vi "Measure_Voltage.vi"(6 "Resolution in Digits":T1(ring), 8 "error in (no error)":errorcluster, 9 "Range":dbl=1.2, 10 "Level":dbl=1.2, 11 "NI-DCPower in":refnum<class "niDCPower.lvclass">) -> (0 "error out":errorcluster, 1 "Out of Range":bool, 2 "DC_Voltage":dbl, 3 "NI-DCPower out":refnum<class "niDCPower.lvclass">)   [LabVIEW 2021, in "niDCPower.lvclass"]
uses:
  niDCPower.lvclass
  <instrlib>/niDCPower/nidcpower.llb/niDCPower Wait For Event - Event.ctl
  <instrlib>/niDCPower/nidcpower.llb/niDCPower Measurement Type.ctl
  niDCPower.lvclass/niDCPower.ctl
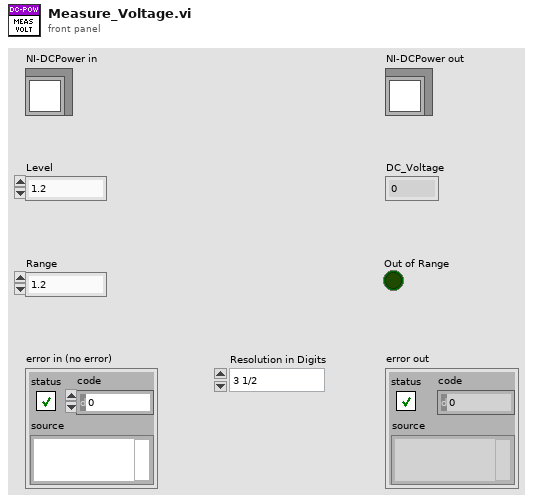
[diagram p1: front panel]
types:
  T1 = enum32{"3 1/2", "4 1/2", "5 1/2", "6 1/2", "7 1/2"}
  T2 = enum32{"DC Volts", "AC Volts", "DC Current", "AC Current", "2-wire Resistance", "4-wire Resistance", "Diode", "Frequency", "Period", "AC Volts DC Coupled", "Capacitance", "Inductance", "Temperature"}
  T3 = typedef "niDCPower Measurement Type.ctl" = i32
  T4 = typedef "niDCPower Wait For Event - Event.ctl" = i32
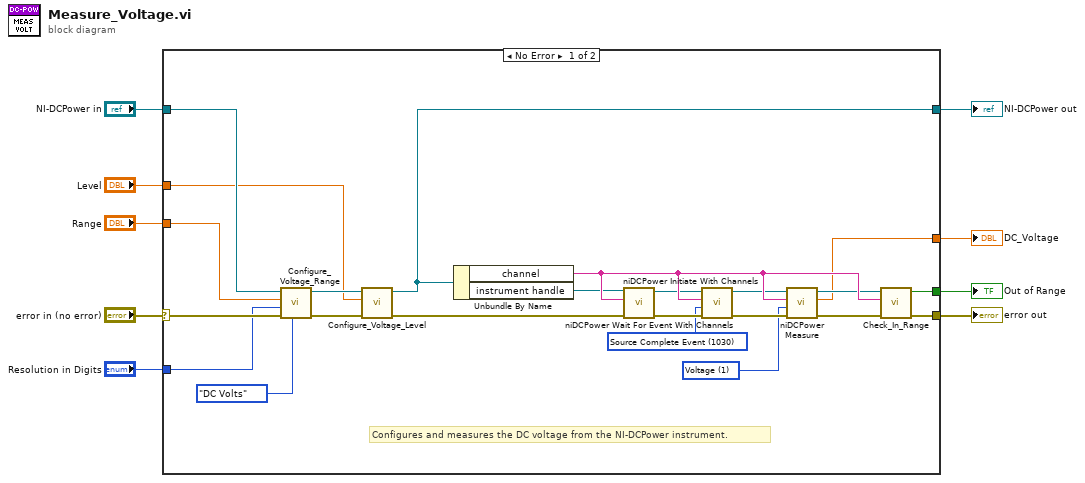
[diagram p0: block diagram]
diagram:
  n1 = case shown="No Error" "error in (no error)" {
    selector: "error in (no error)" -> [w32 w33]
    tunnel: "NI-DCPower in" -> [w13 w34]
    tunnel: [w31 w33] -> w7
    tunnel: [w29 w34] -> w6
    tunnel: "Range" -> [w14 _]
    tunnel: "Resolution in Digits" -> [w15 _]
    tunnel: "Level" -> [w12 _]
    tunnel: [w11 _] -> w2
    tunnel: [w10 _] -> w1
    frame No Error {
      w20 = T3 1 items=["Current", "Voltage"] ("measurement type")
      w24 = T4 1030 items=["Source Complete Event"=1030, "Measure Complete Event"=1031, "Sequence Iteration Complete Event"=1032, "Sequence Engine Done Event"=1033, "Pulse Complete Event"=1051, "Ready For Pulse Trigger Event"=1052] ("event")
      # "Configures and measures the DC voltage from the NI-DCPower instrument."
      n2 = call-dynamic "Configure_Voltage_Range.vi"("Measurement Type"=T2."DC Volts", "error in (no error)"=w32, "Resolution in Digits"=w15, "Range"=w14, "NI-DCPower in"=w13) -> ("error out"=w18:errorcluster, "NI-DCpower out"=w17:refnum<class "niDCPower.lvclass">)  [unwired: 5 in]
      n3 = call-dynamic "Configure_Voltage_Level.vi"("error in (no error)"=w18, "Level"=w12, "niDCPower in"=w17) -> ("error out"=w30:errorcluster, "niDCPower out"=w29:refnum<class "niDCPower.lvclass">)  [unwired: 7 in]
      n4 = Unbundle By Name(w29) -> ("channel"=w28:string, "instrument handle"=w27:refnum<k15>)
      n5 = call <instrlib>:"niDCPower Initiate With Channels.vi"("error in (no error)"=w30, "channel name"=w28, "instrument handle"=w27) -> ("error out"=w25:errorcluster, "instrument handle out"=w26:refnum<k15>)  [unwired: 7 in]
      n6 = call <instrlib>:"niDCPower Wait For Event With Channels.vi"("error in (no error)"=w25, "event"=w24, "channel name"=w28, "instrument handle"=w26) -> ("error out"=w23:errorcluster, "instrument handle out"=w22:refnum<k15>)  [unwired: 6 in]
      n7 = call <instrlib>:"niDCPower Measure.vi"("error in (no error)"=w23, "measurement type"=w20, "channel name"=w28, "instrument handle"=w22) -> ("error out"=w21:errorcluster, "measurement"=w10:dbl, "instrument handle out"=w19:refnum<k15>)  [unwired: 5 in]
      n8 = call "Check_In_Range.vi"("error in (no error)"=w21, "channel name"=w28, "instrument handle"=w19) -> ("error out"=w31:errorcluster, "not in compliance?"=w11:bool)  [unwired: 7 in]
    }
    frame Error {
    }
  }
  "error out" <- w7
  "NI-DCPower out" <- w6
  "DC_Voltage" <- w1
  "Out of Range" <- w2
